vi "Pick&Place_V0.vi"() -> ()   [LabVIEW 2016]
uses:
  Classes/Controllers/I-O/Copy of NI-DAQ Folder/NI-DAQ.lvclass
  Classes/Controllers/Dispenser/Copy of Ultimus V2 Folder/Ultimus V2.lvclass
  <vilib>/Analysis/coordinate.llb/2D Cartesian Coordinate Rotation (Scalar).vi
  <vilib>/Utility/file.llb/Read Delimited Spreadsheet (DBL).vi
  Classes/Controllers/Motion/Copy of Motion Folder/Motion.lvclass
  Classes/Controllers/Camera/Copy of Controller Folder/Controller.lvclass
  <vilib>/Analysis/NI_AALPro.lvlib
panel:
  out "appended array":dbl[](array[numeric])
  out "x-y 2":dbl[][](array[numeric])
  out "Numeric":dbl
  out "element 2":dbl
  out "subarray 2":dbl[](array[numeric])
  out "element":dbl
  in  "Sensor Position":dbl[](array[numeric])=[873.113, 989.0, 47.2259, 0.0]
  in  "Chip tray":dbl[](array[numeric])=[816.244, 706.669, 62.5578, -0.0177741]
  in  "Default top-left\nresidual position":dbl[](array[numeric])=[85.4116, 85.4116, 85.4116, 0.0]
  out "Sample position \non HDI":dbl[][](array[numeric])
  in  "Number of chips\nto be assembled":i32=4
  out "relative position":dbl[](array[numeric])
  out "new relative position":dbl[](array[numeric])
  in  "Continue pick and place? (T)":bool=TRUE
  in  "Measure Chips/Sensor\non sample tray?":bool
  in  "measure pickup tool?":bool
  out "x-y":dbl[](array[numeric])
  in  "If deposit Glue?":bool=TRUE
  in  "DAQ Module 2":i32
  out "Chip Pickup\nTool Central\nPosition":dbl[](array[numeric])
  in  "Chip PickUp\nTool topleft \nposition":dbl[](array[numeric])=[766.263, 963.853, 15.3066, -0.0259463]
  out "ALL Chip position":dbl[][](array[numeric])
  out "chip position":dbl[](array[numeric])
  out "default chip and sensor position w.r.t. 1st mark":dbl[][](array[numeric])
  in  "Assembly Type":bool=TRUE
  out "HDI rotation (rad)":dbl format="%#.6g"
  out "measured distance \nbetween 2 marks\n(ideal 232.6724)":dbl
  out "shift distrance\nof mark 2 w.r.t.\nmark 1":dbl
  out "Between 2 \nmeasured marks":dbl[](array[numeric])
  out "Measured-Default 2":dbl[](array[numeric]) format="%#.3g"
  out "Measured-Default":dbl[](array[numeric]) format="%#.3g"
  out "Measured Residual Mark 2":dbl[](array[numeric])
  out "Measured Residual Mark 1":dbl[](array[numeric])
  # "Chips"
  # "Sensors"
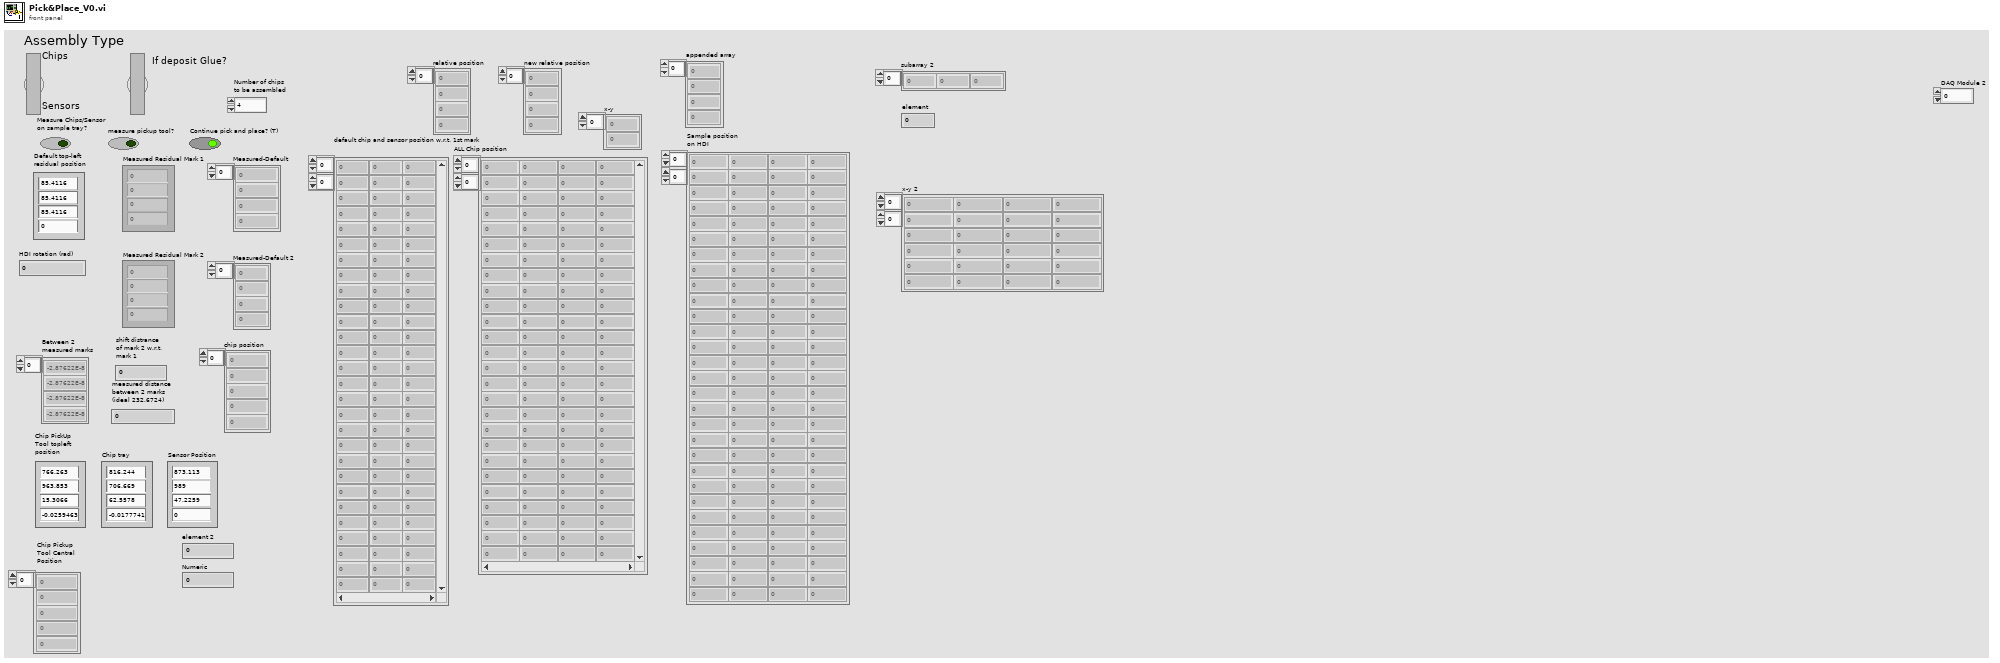
[diagram p1: front panel]
types:
  T1 = typedef "Controller.lvclass/Controllers.ctl" = cluster{"Copy of Motion.lvclass":refnum<class "Motion.lvclass">, "Copy of I-O.lvclass":refnum<class "I-O.lvclass">, "Copy of Dispenser.lvclass":refnum<class "Dispenser.lvclass">}
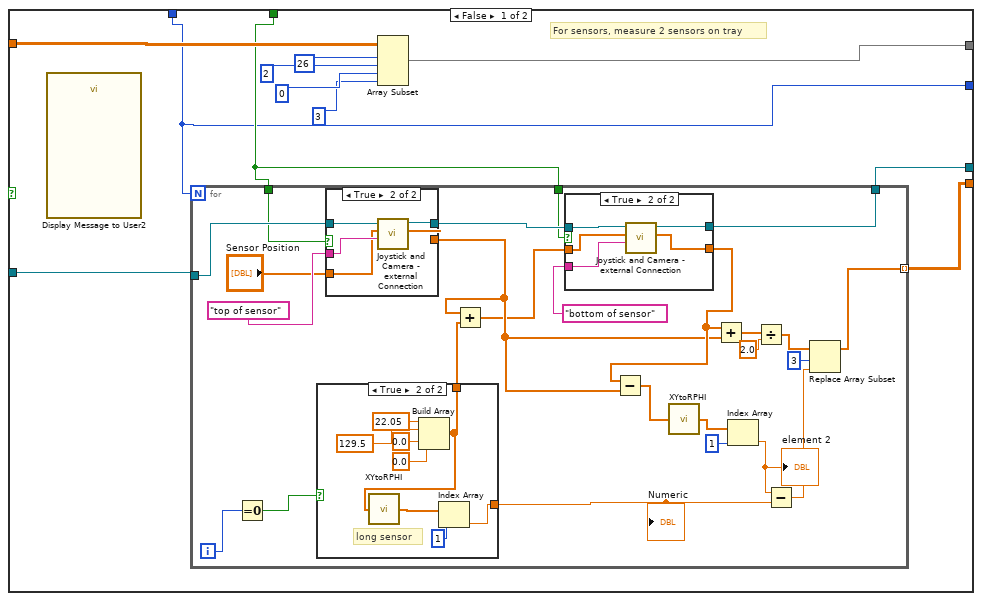
[diagram p2: hidden frame]
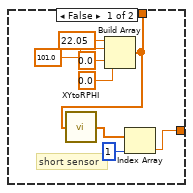
[diagram p3: hidden frame]
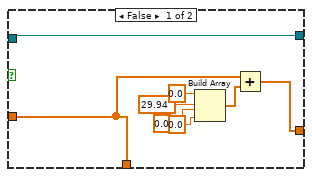
[diagram p8: hidden frame]
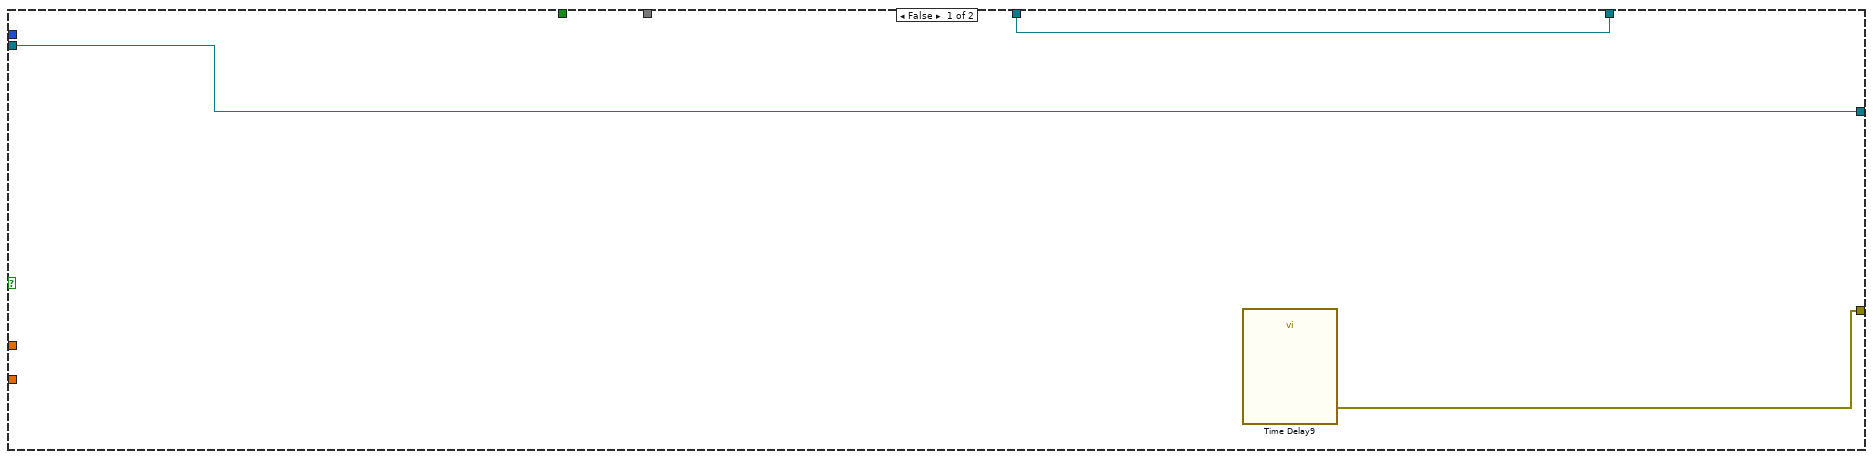
[diagram p9: hidden frame]
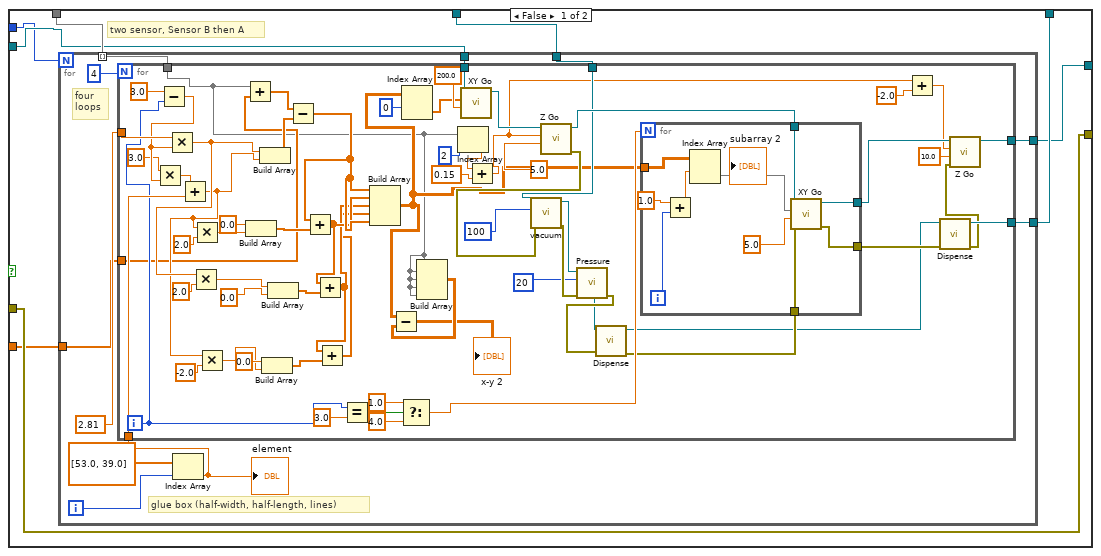
[diagram p10: hidden frame]
diagram:
  w46 = refnum<class "NI-DAQ.lvclass"> refnum  # NI-DAQ.lvclass
  (unwired) "ideal delta Y between \n2 fiducial marks"
  (unwired) "ideal delta X between 2 fiducial marks"
  n1 = flat-sequence {
    tunnel: [w72] -> w61
    tunnel: [w71] -> w60
    tunnel: w57 -> [w77]
    tunnel: [w86] -> w54
    tunnel: w53 -> [w80]
    tunnel: [w66] -> w52
    tunnel: [w72] -> w51
    tunnel: w8 -> [w73]
    tunnel: [w70] -> w7
    tunnel: "Assembly Type" -> [w135]
    tunnel: w61 -> [w133]
    tunnel: w60 -> [w129]
    tunnel: [w134] -> w50
    tunnel: [w133] -> w49
    tunnel: [w130] -> w48
    tunnel: w54 -> [w132]
    tunnel: [w131] -> w47
    tunnel: [w129] -> w34
    tunnel: w7 -> [w128]
    tunnel: [w127] -> w5
    tunnel: w50 -> [w268]
    tunnel: [w268] -> w45
    tunnel: w49 -> [w277]
    tunnel: [w277] -> w44
    tunnel: w48 -> [w276]
    tunnel: [w276] -> w43
    tunnel: w47 -> [w274]
    tunnel: "Assembly Type" -> [w270]
    tunnel: [w275] -> w42
    tunnel: [w273] -> w41
    tunnel: [w272] -> w35
    tunnel: w34 -> [w272]
    tunnel: [w271] -> w6
    tunnel: w5 -> [w271]
    tunnel: w45 -> [w330]
    tunnel: [w330] -> w40
    tunnel: w44 -> [_]
    tunnel: w43 -> [w329]
    tunnel: [w329] -> w39
    tunnel: w42 -> [w333]
    tunnel: [w333] -> w38
    tunnel: w41 -> [w331]
    tunnel: [w328] -> w37
    tunnel: [w327] -> w36
    tunnel: w35 -> [w327]
    tunnel: [w326] -> w30
    tunnel: w24 -> [w325]
    tunnel: [w324] -> w23
    tunnel: w19 -> [w323]
    tunnel: w18 -> [w322]
    tunnel: w6 -> [w321]
    tunnel: [w321] -> w4
    tunnel: "Assembly Type" -> [w320]
    tunnel: w40 -> [w528]
    tunnel: w39 -> [w542]
    tunnel: w38 -> [w539]
    tunnel: [w535] -> w28
    tunnel: "Assembly Type" -> [w529]
    tunnel: w37 -> [w530]
    tunnel: w36 -> [_]
    tunnel: [w534] -> w33
    tunnel: w30 -> [w538]
    tunnel: w26 -> [w531]
    tunnel: w10 -> [w537]
    tunnel: w9 -> [w536]
    tunnel: w4 -> [w533]
    tunnel: w2 -> [w532]
    frame #0 {
      # "MESAURE HDI alignment marks"
      n2 = call "Joystick and Camera - external Connection.vi"("Motion in"=w80, "XYZTheta"="Default top-left\nresidual position", "Measurement Point"="HDI Top-left") -> ("Motion out"=w81:refnum<class "Motion.lvclass">, "Sum"=w74:dbl[], "error out"=w83:errorcluster)  [unwired: 4 in, 1 out]
      "Measured Residual Mark 1" <- w74
      n3 = Subtract(x=w74, y="Default top-left\nresidual position") -> (x-y=→"Measured-Default":dbl[])
      n4 = call "Time Delay3"("error in (no error)"=w83) -> ()  [unwired: 10 in, 1 out]
      n5 = Add(x=w77, y=w74) -> (x+y=w76:dbl[])
      n6 = call "Joystick and Camera - external Connection.vi"("Motion in"=w81, "XYZTheta"=w76, "Measurement Point"="HDI bottom-right") -> ("Motion out"=w86:refnum<class "Motion.lvclass">, "Gantry"=w85:dbl[], "error out"=w84:errorcluster)  [unwired: 4 in, 1 out]
      "Measured Residual Mark 2" <- w85
      n7 = Subtract(x=w85, y=w76) -> (x-y=→"Measured-Default 2":dbl[])
      n8 = Subtract(x=w85, y=w74) -> (x-y=w66:dbl[])
      n9 = call "Time Delay4"("error in (no error)"=w84) -> ()  [unwired: 10 in, 1 out]
      n10 = Index Array(array=w66, index=1) -> (element=w64:dbl)
      n11 = Index Array(array=w66, index=2) -> (element=w68:dbl)
      n12 = call "XYtoRPHI.vi"("X-Y"=w66) -> ("r-phi"=w89:dbl[])
      n13 = Subtract(x=w66, y=w77) -> (x-y=w98:dbl[])
      n14 = call "XYtoRPHI.vi"("X-Y"=w98) -> ("r-phi"=w96:dbl[])
      n15 = call "XYtoRPHI.vi"("X-Y"=w77) -> ("r-phi"=w91:dbl[])
      n16 = Index Array(array=w89, index=1) -> (element=w87:dbl)
      n17 = Index Array(array=w89, index=0) -> (element=→"measured distance \nbetween 2 marks\n(ideal 232.6724)":dbl)
      n18 = Index Array(array=w96, index=0) -> (element=→"shift distrance\nof mark 2 w.r.t.\nmark 1":dbl)
      n19 = Index Array(array=w91, index=1) -> (element=w90:dbl)
      n20 = Subtract(x=w87, y=w90) -> (x-y=w72:dbl)
      n21 = Replace Array Subset(array=w74, new element=w72, index=3) -> (w71:dbl[])
      n22 = for {
        tunnel: w73 -> [w117] mode=indexing
        tunnel: w72 -> [w113]
        tunnel: w71 -> [w106]
        tunnel: [w116] -> w70 mode=indexing
        tunnel: w68 -> [w112]
        tunnel: w64 -> [w103]
        # "Compute  chips/sensor new positions"
        n23 = Index Array(array=w117, index=1) -> (element=w121:dbl)
        n24 = Index Array(array=w117, index=2) -> (element=w120:dbl)
        n25 = Multiply(x=w113, y=-1.0) -> (x*y=w114:dbl)
        n26 = call-poly <vilib>:"2D Cartesian Coordinate Rotation.vi"("theta"=w114, "y"=w120, "x"=w121) -> ("y out"=w123:dbl, "x out"=w122:dbl)  [unwired: 6 in, 1 out]
        n27 = Build Array(w122, w123, 0.0 ("element"), w113) -> (w100:dbl[])
        "new relative position" <- w100
        n28 = Divide(x=w112, y=w103) -> (x/y=w111:dbl)
        n29 = Index Array(array=w100, index=1) -> (element=w101:dbl)
        n30 = Multiply(x=w111, y=w101) -> (x*y=w107:dbl)
        n31 = Build Array(0.0 ("element"), 0.0 ("element"), w107, 0.0 ("element")) -> (w105:dbl[])
        "appended array" <- w105
        n32 = Add(x=w106, y=w105) -> (x+y=w104:dbl[])
        n33 = Add(x=w100, y=w104) -> (x+y=w116:dbl[])
        "relative position" <- w117
      }
      "Sample position \non HDI" <- w70
    }
    frame #1 {
      # "Measure CHIP/SENSOR on sample tray"
      n34 = case shown="True" w135 {
        tunnel: [w136 w202] -> w134
        tunnel: [w138 w207] -> w130
        tunnel: w132 -> [w140 w206]
        tunnel: [w139 w205] -> w131
        tunnel: w128 -> [w142 w204]
        tunnel: [w141 w204] -> w127
        tunnel: "Measure Chips/Sensor\non sample tray?" -> [w137 w203]
        tunnel: "Number of chips\nto be assembled" -> [w136 w202]
        frame False {
          # "For sensors, measure 2 sensors on tray"
          n35 = call "Display Message to User2"() -> ()  [unwired: 10 in, 2 out]
          n36 = for {
            N: w136 -> [_]
            tunnel: w140 -> [w171]
            tunnel: [w167] -> w139
            tunnel: w137 -> [w152]
            tunnel: w137 -> [w151]
            tunnel: [w150] -> w138 mode=indexing
            i -> [w148]
            n37 = Equal To 0?(x=w148) -> (x = 0?=w147:bool)
            n38 = case shown="True" w147 {
              tunnel: [w173 w181] -> w159
              tunnel: [w172 w180] -> w154
              frame False {
                # "short sensor"
                n39 = Build Array(22.05 ("element"), 101.0 ("element"), 0.0 ("element"), 0.0 ("element")) -> (w172:dbl[])
                n40 = call "XYtoRPHI.vi"("X-Y"=w172) -> ("r-phi"=w175:dbl[])
                n41 = Index Array(array=w175, index=1) -> (element=w173:dbl)
              }
              frame True {
                # "long sensor"
                n42 = Build Array(22.05 ("element"), 129.5 ("element"), 0.0 ("element"), 0.0 ("element")) -> (w180:dbl[])
                n43 = call "XYtoRPHI.vi"("X-Y"=w180) -> ("r-phi"=w183:dbl[])
                n44 = Index Array(array=w183, index=1) -> (element=w181:dbl)
              }
            }
            "Numeric" <- w159
            n45 = case shown="True" w152 {
              tunnel: w171 -> [w196 w201]
              tunnel: [w196 w200] -> w168
              tunnel: "top of sensor" -> [_ w198]
              tunnel: [w195 w199] -> w155
              tunnel: "Sensor Position" -> [w195 w197]
              frame False {
              }
              frame True {
                n46 = call "Joystick and Camera - external Connection.vi"("Motion in"=w201, "XYZTheta"=w197, "Measurement Point"=w198) -> ("Motion out"=w200:refnum<class "Motion.lvclass">, "Sum"=w199:dbl[])  [unwired: 4 in, 2 out]
              }
            }
            n47 = Add(x=w155, y=w154) -> (x+y=w153:dbl[])
            n48 = case shown="True" w151 {
              tunnel: w168 -> [w189 w194]
              tunnel: [w188 w191] -> w164
              tunnel: [w189 w193] -> w167
              tunnel: "bottom of sensor" -> [_ w192]
              tunnel: w153 -> [w188 w190]
              frame False {
              }
              frame True {
                n49 = call "Joystick and Camera - external Connection.vi"("Motion in"=w194, "XYZTheta"=w190, "Measurement Point"=w192) -> ("Motion out"=w193:refnum<class "Motion.lvclass">, "Sum"=w191:dbl[])  [unwired: 4 in, 2 out]
              }
            }
            n50 = Subtract(x=w164, y=w155) -> (x-y=w163:dbl[])
            n51 = call "XYtoRPHI.vi"("X-Y"=w163) -> ("r-phi"=w162:dbl[])
            n52 = Add(x=w164, y=w155) -> (x+y=w165:dbl[])
            n53 = Index Array(array=w162, index=1) -> (element=w160:dbl)
            "element 2" <- w160
            n54 = Divide(x=w165, y=2.0) -> (x/y=w158:dbl[])
            n55 = Subtract(x=w160, y=w159) -> (x-y=w157:dbl)
            n56 = Replace Array Subset(array=w158, new element=w157, index=3) -> (w150:dbl[])
          }
          n57 = Array Subset(array=w142, index (row)=26 ("index"), length (row)=2 ("length"), index (col)=0, length (col)=3 ("length")) -> (w141:dbl[][])
        }
        frame True {
          # "For chips, measure 26 chips on tray"
          n58 = call "Display Message to User"() -> ()  [unwired: 10 in, 2 out]
          n59 = for {
            N: w202 -> [_]
            tunnel: [w223] -> w207 mode=indexing
            tunnel: w206 -> [w232]
            tunnel: [w230] -> w205
            tunnel: w203 -> [w222]
            tunnel: w203 -> [w221]
            i -> [w229]
            n60 = Quotient & Remainder(x=w229, y=4) -> (x-y*floor(x/y)=w248:i32, floor(x/y)=w250:i32)
            n61 = Number To Decimal String(number=w229, width (-)=i16 2) -> (decimal integer string=w227:string)
            n62 = Multiply(x=w250, y=-5) -> (x*y=w247:i32)
            n63 = Concatenate Strings("Top left of Chip  " ("string"), w227) -> (w219:string)
            n64 = Multiply(x=w248, y=11.15) -> (x*y=w246:dbl)
            n65 = Build Array(w247, w246, 0.0 ("element"), 0.0 ("element")) -> (w245:dbl[])
            n66 = Add(x="Chip tray", y=w245) -> (x+y=w242:dbl[])
            n67 = case shown="True" w222 {
              tunnel: w232 -> [w260 w266]
              tunnel: [w260 w265] -> w231
              tunnel: w242 -> [w261 w264]
              tunnel: w219 -> [_ w263]
              tunnel: [w261 w262] -> w226
              frame False {
              }
              frame True {
                n68 = call "Joystick and Camera - external Connection.vi"("Motion in"=w266, "XYZTheta"=w264, "Measurement Point"=w263) -> ("Motion out"=w265:refnum<class "Motion.lvclass">, "Sum"=w262:dbl[])  [unwired: 4 in, 2 out]
              }
            }
            n69 = Concatenate Strings("Bottom right of Chip  " ("string"), w227) -> (w216:string)
            n70 = Build Array(2.64 ("element"), 9.09 ("element"), 0.0 ("element"), 0.0 ("element")) -> (w212:dbl[])
            n71 = Add(x=w226, y=w212) -> (x+y=w218:dbl[])
            n72 = case shown="True" w221 {
              tunnel: w231 -> [w253 w259]
              tunnel: w218 -> [w254 w258]
              tunnel: [w254 w255] -> w233
              tunnel: [w253 w257] -> w230
              tunnel: w216 -> [_ w256]
              frame False {
              }
              frame True {
                n73 = call "Joystick and Camera - external Connection.vi"("Motion in"=w259, "XYZTheta"=w258, "Measurement Point"=w256) -> ("Motion out"=w257:refnum<class "Motion.lvclass">, "Sum"=w255:dbl[])  [unwired: 4 in, 2 out]
              }
            }
            n74 = Subtract(x=w233, y=w226) -> (x-y=w215:dbl[])
            n75 = call "XYtoRPHI.vi"("X-Y"=w212) -> ("r-phi"=w214:dbl[])
            n76 = Add(x=w226, y=w233) -> (x+y=w240:dbl[])
            n77 = call "XYtoRPHI.vi"("X-Y"=w215) -> ("r-phi"=w237:dbl[])
            n78 = Index Array(array=w214, index=1) -> (element=w209:dbl)
            n79 = Divide(x=w240, y=2.0) -> (x/y=w225:dbl[])
            n80 = Index Array(array=w237, index=1) -> (element=w210:dbl)
            n81 = Subtract(x=w210, y=w209) -> (x-y=w211:dbl)
            n82 = Replace Array Subset(array=w225, new element=w211, index=3) -> (w223:dbl[])
            "chip position" <- w223
          }
        }
      }
      "ALL Chip position" <- w130
    }
    frame #2 {
      # "Measure PIckupTool"
      n83 = Select(t=1.0, s=w270, f=w268) -> (s? t:f=w267:dbl)
      n84 = for {
        N: w267 -> [_]
        tunnel: [w284] -> w275 mode=indexing
        tunnel: w274 -> [w291]
        tunnel: [w290] -> w273
        # "Default size and\norientation"
        n85 = case shown="True" "measure pickup tool?" {
          tunnel: w291 -> [w305 w306]
          tunnel: [w305 w308] -> w290
          tunnel: "Chip PickUp\nTool topleft \nposition" -> [w301 w307]
          tunnel: [w301 w311] -> w288
          tunnel: [w300 w310] -> w287
          frame False {
            n86 = Build Array(0.0 ("element"), 29.94 ("element"), 0.0 ("element"), 0.0 ("element")) -> (w304:dbl[])
            n87 = Add(x=w301, y=w304) -> (x+y=w300:dbl[])
          }
          frame True {
            n88 = call "Joystick and Camera - external Connection.vi"("Motion in"=w306, "XYZTheta"=w307, "Measurement Point"="PickUp tool TopLeft") -> ("Motion out"=w309:refnum<class "Motion.lvclass">, "Sum"=w311:dbl[])  [unwired: 4 in, 2 out]
            n89 = Build Array(0.0 ("element"), 29.94 ("element"), 0.0 ("element"), 0.0 ("element")) -> (w317:dbl[])
            n90 = Add(x=w311, y=w317) -> (x+y=w312:dbl[])
            n91 = call "Joystick and Camera - external Connection.vi"("Motion in"=w309, "XYZTheta"=w312, "Measurement Point"="PickUp tool BottomRight") -> ("Motion out"=w308:refnum<class "Motion.lvclass">, "Sum"=w310:dbl[])  [unwired: 4 in, 2 out]
          }
        }
        n92 = Add(x=w288, y=w287) -> (x+y=w296:dbl[])
        n93 = Subtract(x=w287, y=w288) -> (x-y=w285:dbl[])
        n94 = Divide(x=w296, y=2.0) -> (x/y=w293:dbl[])
        n95 = call "XYtoRPHI.vi"("X-Y"=w285) -> ("r-phi"=w294:dbl[])
        n96 = Index Array(array=w294, index=1) -> (element=w279:dbl)
        n97 = Absolute Value(x=w279) -> (abs(x)=w282:dbl)
        n98 = Sign(1:w279) -> (0:w280:dbl)
        n99 = Subtract(x=w282, y=1.5707963267948966) -> (x-y=w281:dbl)
        n100 = Multiply(x=w280, y=w281) -> (x*y=w278:dbl)
        n101 = Replace Array Subset(array=w293, new element=w278, index=3) -> (w284:dbl[])
        "Chip Pickup\nTool Central\nPosition" <- w284
      }
    }
    frame #3 {
      # "If deposit glue"
      n102 = case shown="True" "If deposit Glue?" {
        tunnel: w327 -> [_ w380]
        tunnel: w331 -> [w336 w378]
        tunnel: w330 -> [_ w368]
        tunnel: [w336 w366] -> w328
        tunnel: w327 -> [_ w356]
        tunnel: [w335 w364] -> w326
        tunnel: w325 -> [w334 w352]
        tunnel: [w334 w351] -> w324
        tunnel: w323 -> [_ w348]
        tunnel: w322 -> [_ w347]
        tunnel: w321 -> [_ w346]
        tunnel: w320 -> [_ w337]
        frame False {
          n103 = call "Time Delay9"() -> ("error out"=w335:errorcluster)  [unwired: 11 in]
        }
        frame True {
          # "Unmount syringe"
          # "parking position away from \n1st alignment mark (Z value\nrepresent glue gap)"
          # "Syringe-camera offset"
          n104 = Build Array(w348, w347, 0.0 ("element"), 0.0 ("element")) -> (w367:dbl[])
          n105 = Build Array(11.75, -25, 0.5 ("element"), 0.0 ("element")) -> (w375:dbl[])
          n106 = Add(x=w367, y=w375) -> (x+y=w370:dbl[])
          n107 = Add(x=w380, y=w370) -> (x+y=w379:dbl[])
          n108 = call "XYZTheta Go.vi"("XYZTheta In"=w379, "Motion in"=w378) -> ("error out"=w369:errorcluster, "XYZTheta Out"=w360:dbl[], "Motion out"=w344:refnum<class "Motion.lvclass">)  [unwired: 7 in]
          n109 = call "Display Message to User4"("error in (no error)"=w369) -> ("error out"=w340:errorcluster)  [unwired: 9 in, 1 out]
          n110 = Index Array(array=w360, index=2) -> (element=w345:dbl)
          n111 = call-dynamic "Z Go.vi"("error in (no error)"=w340, "Speed"=20.0, "Position"=0.0, "Motion in"=w344) -> ("error out"=w339:errorcluster, "Motion out"=w343:refnum<class "Motion.lvclass">)  [unwired: 6 in]
          n112 = Add(x=w345, y=-2.5) -> (x+y=w353:dbl)
          n113 = call "Display Message to User5"("error in (no error)"=w339) -> ("error out"=w338:errorcluster)  [unwired: 9 in, 1 out]
          n114 = call-dynamic "Z Go.vi"("error in (no error)"=w338, "Speed"=20.0, "Position"=w353, "Motion in"=w343) -> ("error out"=w362:errorcluster, "Motion out"=w363:refnum<class "Motion.lvclass">)  [unwired: 6 in]
          n115 = case shown="True" w337 {
            tunnel: w368 -> [w381 w484]
            tunnel: w367 -> [w382 w483]
            tunnel: w363 -> [w386 w482]
            tunnel: w362 -> [w387 w481]
            tunnel: w352 -> [w385 w480]
            tunnel: [w384 w479] -> w351
            tunnel: [w383 w478] -> w350
            tunnel: [w387 w477] -> w349
            tunnel: w346 -> [w388 w476]
            frame False {
              # "two sensor, Sensor B then A"
              n116 = for {
                N: w381 -> [_]
                tunnel: w388 -> [w396] mode=indexing
                tunnel: w386 -> [w393]
                tunnel: w385 -> [w392]
                tunnel: [w391] -> w384
                tunnel: [w390] -> w383
                tunnel: w382 -> [w389]
                i -> [w398]
                # "four\nloops"
                # "glue box (half-width, half-length, lines)"
                n117 = Index Array(array=dbl[] [53.0, 39.0], index=w398) -> (element=w394:dbl)
                "element" <- w394
                n118 = for {
                  N: 4 -> [_]
                  tunnel: w396 -> [w405]
                  tunnel: 2.81 -> [w464]
                  tunnel: w394 -> [w456]
                  tunnel: w393 -> [w436]
                  tunnel: w392 -> [w417]
                  tunnel: [w416] -> w391
                  tunnel: [w411] -> w390
                  tunnel: w389 -> [w408]
                  i -> [w426]
                  n119 = Subtract(x=3.0, y=w426) -> (x-y=w463:dbl)
                  n120 = Multiply(x=3.0, y=w463) -> (x*y=w457:dbl)
                  n121 = Multiply(x=w464, y=w463) -> (x*y=w452:dbl)
                  n122 = Add(x=w457, y=w456) -> (x+y=w450:dbl)
                  n123 = Multiply(x=w452, y=2.0) -> (x*y=w453:dbl)
                  n124 = Multiply(x=w450, y=2.0) -> (x*y=w459:dbl)
                  n125 = Multiply(x=w450, y=-2.0) -> (x*y=w449:dbl)
                  n126 = Add(x=w405, y=w408) -> (x+y=w407:dbl[])
                  n127 = Build Array(0.0 ("element"), w459) -> (w447:dbl[])
                  n128 = Build Array(w452, w450) -> (w448:dbl[])
                  n129 = Build Array(0.0 ("element"), w449) -> (w445:dbl[])
                  n130 = Build Array(w453, 0.0 ("element")) -> (w446:dbl[])
                  n131 = Subtract(x=w407, y=w448) -> (x-y=w444:dbl[])
                  n132 = Add(x=w444, y=w447) -> (x+y=w443:dbl[])
                  n133 = Add(x=w443, y=w446) -> (x+y=w442:dbl[])
                  n134 = Add(x=w442, y=w445) -> (x+y=w441:dbl[])
                  n135 = Equal?(x=w426, y=3.0) -> (x = y?=w425:bool)
                  n136 = Build Array(w444, w443, w442, w441, w444) -> (w406:dbl[][])
                  n137 = Select(t=1.0, s=w425, f=4.0) -> (s? t:f=w422:dbl)
                  n138 = Index Array(array=w406, index (row)=0) -> (element=w439:dbl[])  [unwired: 1 in]
                  n139 = Build Array(w405, w405, w405, w405, w405) -> (w404:dbl[][])
                  n140 = Subtract(x=w406, y=w404) -> (x-y=→"x-y 2":dbl[][])
                  n141 = Index Array(array=w405, index=2) -> (element=w401:dbl)
                  n142 = call-dynamic "XY Go.vi"("Speed"=200.0, "XY"=w439, "Motion in"=w436) -> ("Motion out"=w435:refnum<class "Motion.lvclass">)  [unwired: 7 in, 1 out]
                  n143 = Add(x=w401, y=0.15) -> (x+y=w400:dbl)
                  n144 = call-dynamic "Z Go.vi"("Speed"=5.0, "Position"=w400, "Motion in"=w435) -> ("error out"=w428:errorcluster, "Motion out"=w421:refnum<class "Motion.lvclass">)  [unwired: 7 in]
                  n145 = call "vacuum.vi"("error in (no error)"=w428, "Vacuum Setting (0000)"=i64 100, "Ultimus V in"=w417) -> ("error out"=w433:errorcluster, "Ultimus V out"=w431:refnum<class "Ultimus V2.lvclass">)  [unwired: 7 in]
                  n146 = call-dynamic "Pressure.vi"("error in (no error)"=w433, "Pressure"=i16 20, "Ultimus V in"=w431) -> ("error out"=w434:errorcluster, "Ultimus V out"=w429:refnum<class "Ultimus V2.lvclass">)  [unwired: 7 in]
                  n147 = call-dynamic "Dispense.vi"("error in (no error)"=w434, "Ultimus V in"=w429) -> ("error out"=w420:errorcluster, "Ultimus V out"=w418:refnum<class "Ultimus V2.lvclass">)  [unwired: 8 in]
                  n148 = for {
                    N: w422 -> [_]
                    tunnel: w406 -> [w474]
                    tunnel: w421 -> [w470]
                    tunnel: w420 -> [w469]
                    tunnel: [w468] -> w419
                    tunnel: [w467] -> w415
                    i -> [w472]
                    n149 = Add(x=1.0 ("y"), y=w472) -> (x+y=w466:dbl)
                    n150 = Index Array(array=w474, index (row)=w466) -> (element=w471:dbl[])  [unwired: 1 in]
                    "subarray 2" <- w471
                    n151 = call-dynamic "XY Go.vi"("error in (no error)"=w469, "Speed"=5.0, "XY"=w471, "Motion in"=w470) -> ("error out"=w468:errorcluster, "Motion out"=w467:refnum<class "Motion.lvclass">)  [unwired: 6 in]
                  }
                  n152 = Add(x=w400, y=-2.0) -> (x+y=w412:dbl)
                  n153 = call-dynamic "Dispense.vi"("error in (no error)"=w419, "Ultimus V in"=w418) -> ("error out"=w410:errorcluster, "Ultimus V out"=w416:refnum<class "Ultimus V2.lvclass">)  [unwired: 8 in]
                  n154 = call-dynamic "Z Go.vi"("error in (no error)"=w410, "Speed"=10.0, "Position"=w412, "Motion in"=w415) -> ("Motion out"=w411:refnum<class "Motion.lvclass">)  [unwired: 6 in, 1 out]
                }
              }
            }
            frame True {
              n155 = for {
                N: w484 -> [_]
                tunnel: w482 -> [w520]
                tunnel: w481 -> [w519]
                tunnel: w483 -> [w518]
                tunnel: w480 -> [w503]
                tunnel: [w502] -> w479
                tunnel: [w501] -> w478
                tunnel: [w500] -> w477
                tunnel: w476 -> [w487] mode=indexing
                n156 = Index Array(array=w487, index=2) -> (element=w489:dbl)
                n157 = Add(x=w489, y=0.37) -> (x+y=w488:dbl)
                n158 = Add(x=w487, y=w518) -> (x+y=w517:dbl[])
                n159 = Build Array(-0.1 ("element"), 3.0 ("element")) -> (w524:dbl[])
                n160 = Subtract(x=w517, y=w524) -> (x-y=w525:dbl[])
                "x-y" <- w525
                n161 = Add(x=w517, y=w524) -> (x+y=w498:dbl[])
                n162 = call-dynamic "XY Go.vi"("error in (no error)"=w519, "Speed"=200.0, "XY"=w525, "Motion in"=w520) -> ("error out"=w504:errorcluster, "Motion out"=w496:refnum<class "Motion.lvclass">)  [unwired: 6 in]
                n163 = call-dynamic "Z Go.vi"("error in (no error)"=w504, "Speed"=5.0, "Position"=w488, "Motion in"=w496) -> ("error out"=w486:errorcluster)  [unwired: 6 in, 1 out]
                n164 = call "Display Message to User7"("error in (no error)"=w486) -> ("error out"=w485:errorcluster)  [unwired: 9 in, 1 out]
                n165 = call "vacuum.vi"("error in (no error)"=w485, "Vacuum Setting (0000)"=i64 100, "Ultimus V in"=w503) -> ("error out"=w514:errorcluster, "Ultimus V out"=w509:refnum<class "Ultimus V2.lvclass">)  [unwired: 7 in]
                n166 = call-dynamic "Pressure.vi"("error in (no error)"=w514, "Pressure"=i16 20, "Ultimus V in"=w509) -> ("error out"=w515:errorcluster, "Ultimus V out"=w506:refnum<class "Ultimus V2.lvclass">)  [unwired: 7 in]
                n167 = call-dynamic "Dispense.vi"("error in (no error)"=w515, "Ultimus V in"=w506) -> ("error out"=w497:errorcluster, "Ultimus V out"=w505:refnum<class "Ultimus V2.lvclass">)  [unwired: 8 in]
                n168 = call "Time Delay6"("error in (no error)"=w497) -> ("error out"=w495:errorcluster)  [unwired: 10 in]
                n169 = call-dynamic "XY Go.vi"("error in (no error)"=w495, "Speed"=5.0, "XY"=w498, "Motion in"=w496) -> ("error out"=w494:errorcluster, "Motion out"=w492:refnum<class "Motion.lvclass">)  [unwired: 6 in]
                n170 = call "Time Delay12"("error in (no error)"=w494) -> ("error out"=w493:errorcluster)  [unwired: 10 in]
                n171 = call "Time Delay10"("error in (no error)"=w495) -> ("error out"=w508:errorcluster)  [unwired: 10 in]
                n172 = call-dynamic "Dispense.vi"("error in (no error)"=w508, "Ultimus V in"=w505) -> ("Ultimus V out"=w502:refnum<class "Ultimus V2.lvclass">)  [unwired: 8 in, 1 out]
                n173 = Add(x=w488, y=-2.5) -> (x+y=w512:dbl)
                n174 = call-dynamic "Z Go.vi"("error in (no error)"=w493, "Speed"=10.0, "Position"=w512, "Motion in"=w492) -> ("error out"=w500:errorcluster, "Motion out"=w501:refnum<class "Motion.lvclass">)  [unwired: 6 in]
              }
            }
          }
          n175 = Replace Array Subset(array=w356, new element=0.0 ("new element/subarray"), index=2) -> (w355:dbl[])
          n176 = call "XYZTheta Go.vi"("error in (no error)"=w349, "XYZTheta In"=w355, "Motion in"=w350) -> ("error out"=w365:errorcluster, "Motion out"=w366:refnum<class "Motion.lvclass">)  [unwired: 6 in, 1 out]
          n177 = call "Display Message to User3"("error in (no error)"=w365) -> ("error out"=w364:errorcluster)  [unwired: 9 in, 1 out]
        }
      }
    }
    frame #4 {
      n178 = Not(x="Continue pick and place? (T)") -> (.not. x?=w526:bool)
      n179 = Select(t=1.0, s=w529, f=w528) -> (s? t:f=w540:dbl)
      n180 = Stop(stop? (T)=w526) -> ()
      n181 = for {
        N: w540 -> [_]
        tunnel: w528 -> [w557]
        tunnel: w542 -> [w553]
        tunnel: w530 -> [w593]
        tunnel: [w569] -> w535
        tunnel: w539 -> [w591] mode=indexing
        tunnel: [w576] -> w534
        tunnel: w538 -> [w588]
        tunnel: w531 -> [w575]
        tunnel: w537 -> [w574]
        tunnel: w536 -> [w573]
        tunnel: w533 -> [w550]
        tunnel: w532 -> [w568]
        tunnel: w529 -> [w549]
        i -> [w547]
        # "A long\nsensor"
        # "B short \nsensor"
        # "chip pickup tool"
        # "pickup too height offset"
        # "Pick up PICKUP TOOL"
        # "Pick up CHIPs/Sensor and place on HDI"
        n182 = Select(t=w557, s=w549, f=1) -> (s? t:f=w556:i32)
        n183 = Equal?(x=w547, y=0) -> (x = y?=w561:bool)
        n184 = Build Array(w574, w573, w568, 0.0 ("element")) -> (w566:dbl[])
        n185 = Add(x=w591, y=w566) -> (x+y=w567:dbl[])
        n186 = call "XYZTheta-2Zspeed Go.vi"("error in (no error)"=w588, "XYZTheta In"=w567, "Motion in"=w593) -> ("error out"=w594:errorcluster, "Motion out"=w592:refnum<class "Motion.lvclass">)  [unwired: 6 in, 1 out]
        n187 = Select(t=-13.7073 ("f"), s=w561, f=-13.2481 ("t")) -> (s? t:f=w559:dbl)
        n188 = Select(t=-21.3804 ("new element/subarray"), s=w549, f=w559) -> (s? t:f=w558:dbl)
        n189 = call-dynamic "Digital Write Multiple Channels.vi"("DAQ Module"="DAQ Module 2", "error in (no error)"=w594, "Values"=bool[] [TRUE] ("values 4"), "Indices"=i32[] [1] ("indices 2"), "NI-DAQ in"=w575) -> ("error out"=w595:errorcluster, "NI-DAQ out"=w571:refnum<class "NI-DAQ.lvclass">)  [unwired: 5 in]
        n190 = Index Array(array=w553, index (row)=w547) -> (element=w552:dbl[])  [unwired: 1 in]
        n191 = Replace Array Subset(array=w566, new element=w558, index=2) -> (w564:dbl[])
        n192 = call "Time Delay7"("error in (no error)"=w595) -> ("error out"=w589:errorcluster)  [unwired: 10 in]
        n193 = Build Array(w552, w552) -> (w551:dbl[][])
        n194 = Select(t=w553, s=w549, f=w551) -> (s? t:f=w554:dbl[][])
        n195 = Index Array(array=w550, index (row)=w547) -> (element=w548:dbl[])  [unwired: 1 in]
        n196 = Build Array(w548, w548) -> (w545:dbl[][])
        n197 = Select(t=w550, s=w549, f=w545) -> (s? t:f=w546:dbl[][])
        n198 = for {
          N: w556 -> [_]
          tunnel: w554 -> [w607] mode=indexing
          tunnel: w592 -> [w609]
          tunnel: w564 -> [w608]
          tunnel: w589 -> [w606]
          tunnel: [w605] -> w577
          tunnel: "DAQ Module 2" -> [w604]
          tunnel: w571 -> [w603]
          tunnel: [w600] -> w570
          tunnel: w546 -> [w599] mode=indexing
          tunnel: [w598] -> w563
          n199 = flat-sequence {
            tunnel: w607 -> [w622]
            tunnel: [w625] -> w610
            tunnel: w609 -> [w623]
            tunnel: w608 -> [w621]
            tunnel: w606 -> [w619]
            tunnel: w604 -> [w618]
            tunnel: w603 -> [w617]
            tunnel: [w612] -> w602
            tunnel: [w613] -> w601
            tunnel: w610 -> [w647]
            tunnel: [w646] -> w605
            tunnel: [w645] -> _
            tunnel: w608 -> [w638]
            tunnel: w602 -> [w641]
            tunnel: w601 -> [w640]
            tunnel: [w639] -> w600
            tunnel: w599 -> [w637]
            tunnel: [w635] -> w598
            frame #0 {
              # "pickup sample from tray"
              n200 = Add(x=w622, y=w621) -> (x+y=w620:dbl[])
              n201 = call "XYZTheta-2Zspeed Go.vi"("error in (no error)"=w619, "XYZTheta In"=w620, "Motion in"=w623) -> ("error out"=w624:errorcluster, "Motion out"=w625:refnum<class "Motion.lvclass">)  [unwired: 6 in, 1 out]
              n202 = call "Time Delay"("error in (no error)"=w624) -> ("error out"=w616:errorcluster)  [unwired: 10 in]
              n203 = call-dynamic "Digital Write Multiple Channels.vi"("DAQ Module"=w618, "error in (no error)"=w616, "Values"=bool[] [TRUE], "Indices"=i32[] [0], "NI-DAQ in"=w617) -> ("error out"=w611:errorcluster, "NI-DAQ out"=w613:refnum<class "NI-DAQ.lvclass">)  [unwired: 5 in]
              n204 = call "Time Delay13"("error in (no error)"=w611) -> ("error out"=w612:errorcluster)  [unwired: 10 in]
            }
            frame #1 {
              # "lift for chip/sensor thickness"
              # "place sample on HDI"
              n205 = Add(x=w637, y=w638) -> (x+y=w630:dbl[])
              n206 = Build Array(0.0 ("element"), 0.0 ("element"), -0.65 ("element"), 0.0 ("element")) -> (w629:dbl[])
              n207 = Add(x=w630, y=w629) -> (x+y=w628:dbl[])
              n208 = call "XYZTheta-2Zspeed Go.vi"("error in (no error)"=w641, "XYZTheta In"=w628, "Motion in"=w647) -> ("error out"=w627:errorcluster, "XYZTheta Out"=w645:dbl[], "Motion out"=w646:refnum<class "Motion.lvclass">)  [unwired: 6 in]
              n209 = call "Display Message to User6"("error in (no error)"=w627) -> ("error out"=w626:errorcluster)  [unwired: 9 in, 1 out]
              n210 = call "Time Delay2"("error in (no error)"=w626) -> ("error out"=w643:errorcluster)  [unwired: 10 in]
              n211 = call-dynamic "Digital Write Multiple Channels.vi"("error in (no error)"=w643, "Values"=bool[] [FALSE], "Indices"=i32[] [0], "NI-DAQ in"=w640) -> ("error out"=w636:errorcluster, "NI-DAQ out"=w639:refnum<class "NI-DAQ.lvclass">)  [unwired: 6 in]
              n212 = call "Time Delay11"("error in (no error)"=w636) -> ("error out"=w635:errorcluster)  [unwired: 10 in]
            }
          }
        }
        n213 = call "XYZTheta-2Zspeed Go.vi"("error in (no error)"=w563, "XYZTheta In"=w567, "Motion in"=w577) -> ("error out"=w583:errorcluster, "Motion out"=w581:refnum<class "Motion.lvclass">)  [unwired: 6 in, 1 out]
        n214 = call "Time Delay5"("error in (no error)"=w583) -> ("error out"=w584:errorcluster)  [unwired: 10 in]
        n215 = call-dynamic "Digital Write Multiple Channels.vi"("DAQ Module"=0, "error in (no error)"=w584, "Values"=bool[] [FALSE], "Indices"=i32[] [1], "NI-DAQ in"=w570) -> ("error out"=w582:errorcluster, "NI-DAQ out"=w576:refnum<class "NI-DAQ.lvclass">)  [unwired: 5 in]
        n216 = call "Time Delay8"("error in (no error)"=w582) -> ("error out"=w578:errorcluster)  [unwired: 10 in]
        n217 = call-dynamic "Z Go.vi"("error in (no error)"=w578, "Speed"=10.0, "Position"=10.0 ("new element/subarray"), "Motion in"=w581) -> ("Motion out"=w569:refnum<class "Motion.lvclass">)  [unwired: 6 in, 1 out]
      }
    }
  }
  n218 = call "Obtain Control Cluster.vi"("I/O"=FALSE) -> ("Control Out"=w55:T1)  [unwired: 10 in]
  n219 = Unbundle By Name(w55) -> ("Copy of Motion.lvclass"=w53:refnum<class "Motion.lvclass">)
  n220 = Build Array(24.3 ("y"), 231.4 ("y"), -0.05 ("element"), 0.0 ("element")) -> (w57:dbl[])
  n221 = call-poly <vilib>:"Read Delimited Spreadsheet.vi"("file path (dialog if empty)"=path "D:/INTT/V1/tmp.txt", "number of rows (all:-1)"=-1) -> ("all rows"=w8:dbl[][])  [unwired: 8 in, 5 out]
  "default chip and sensor position w.r.t. 1st mark" <- w8
  n222 = call-poly <vilib>:"Read Delimited Spreadsheet.vi"("file path (dialog if empty)"=path "D:/INTT/V1/Assembly Data/Tool Offsets/Dispense Tip Offset.txt", "number of rows (all:-1)"=-1) -> ("first row"=w20:dbl[])  [unwired: 8 in, 5 out]
  n223 = Index Array(array=w20, index #1=0 ("index"), index #2=1 ("index")) -> (element #1=w19:dbl, element #2=w18:dbl)
  n224 = call-dynamic "Connect.vi"("Ultimus V in"=refnum<class "Ultimus V2.lvclass"> refnum ("Ultimus V2.lvclass")) -> ("Ultimus V out"=w24:refnum<class "Ultimus V2.lvclass">)  [unwired: 9 in, 1 out]
  n225 = call-dynamic "Disconnect.vi"("Ultimus V in"=w23) -> ()  [unwired: 9 in, 1 out]
  n226 = call-poly <vilib>:"Read Delimited Spreadsheet.vi"("file path (dialog if empty)"=path "D:/INTT/V1/Assembly Data/Tool Offsets/Bellows Tool Offset.txt", "number of rows (all:-1)"=-1) -> ("first row"=w13:dbl[])  [unwired: 8 in, 5 out]
  n227 = Index Array(array=w13, index #1=0 ("index"), index #2=1 ("index"), index #3=2 ("index")) -> (element #1=w10:dbl, element #2=w9:dbl, element #3=w2:dbl)
  n228 = call-dynamic "Connect.vi"("NI-DAQ in"=w46) -> ("NI-DAQ out"=w26:refnum<class "NI-DAQ.lvclass">)  [unwired: 9 in, 1 out]
  n229 = call "XYZTheta Go.vi"("XYZTheta In"=dbl[] [625.0, 625.0], "Motion in"=w28) -> ("Motion out"=w27:refnum<class "Motion.lvclass">)  [unwired: 7 in, 2 out]
  n230 = call-dynamic "Disconnect.vi"("Controller in"=w27) -> ()  [unwired: 9 in, 1 out]
  n231 = call-dynamic "Disconnect.vi"("I-O in"=w33) -> ()  [unwired: 9 in, 1 out]
  "Between 2 \nmeasured marks" <- w52
  "HDI rotation (rad)" <- w51
